vi "LoadConnectionIDerror.vi"(8 "ArrayIN":T1(array[cluster])=[{"IPaddress"="127.0.0.1", "Port"=63400, "connection ID"=refnum, "TCP error"={"status"=TRUE, "code"=1, "source"="TCP Write in TCPwrite8bytesMC.vi->PicoCmdClientMOVE-ForMasterControl_3.vi->Manual command_11.vi"}}], 9 "ErrorIn":errorcluster, 11 "index":i32) -> (0 "ArrayOUT":T1(array[cluster])=[{"IPaddress"="127.0.0.1", "Port"=63400, "connection ID"=refnum, "TCP error"={"status"=TRUE, "code"=1, "source"="TCP Write in TCPwrite8bytesMC.vi->PicoCmdClientMOVE-ForMasterControl_3.vi->Manual command_11.vi"}}])   [LabVIEW 2013]
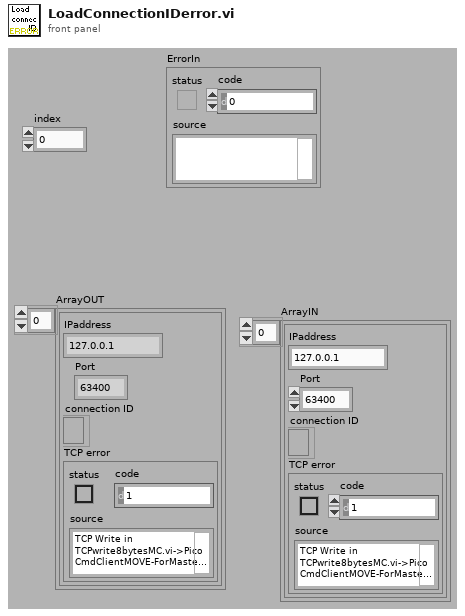
[diagram p1: front panel]
types:
  T1 = cluster{"IPaddress":string, "Port":i32, "connection ID":refnum<k5>, "TCP error":errorcluster}[]
  T2 = cluster{"IPaddress":string, "Port":i32, "connection ID":refnum<k5>, "TCP error":errorcluster}
  T3 = cluster{"IPaddress":string, "Port":i32, "connection ID":refnum<k5>, "ErrorIn":errorcluster}
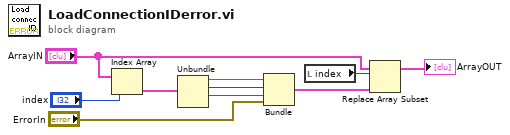
[diagram p0: block diagram]
diagram:
  n1 = Index Array(array="ArrayIN", index="index") -> (element=w9:T2)
  n2 = Unbundle(w9) -> ("IPaddress"=w8:string, "Port"=w7:i32, "connection ID"=w6:refnum<k5>)  [unwired: 1 out]
  n3 = Bundle("IPaddress"=w8, "Port"=w7, "connection ID"=w6, "ErrorIn"="ErrorIn") -> (w4:T3)  [unwired: 1 out]
  n4 = local read "index"() -> (w3:i32)
  n5 = Replace Array Subset(array="ArrayIN", new element=w4, index=w3) -> (→"ArrayOUT":T1)
